vi "LaserLineDetection_Intensity_Imax.vi"(6 "Color":u32(colorbox)=16744448, 8 "error in (no error)":errorcluster, 10 "Line Coordinates":i32[](array[numeric]), 11 "Image In":T2) -> (0 "error out":errorcluster, 1 "appended array":cluster{u8[], i32[]}[](array[cluster]), 2 "Point Information":T1, 3 "Image Out":T2)   [LabVIEW 2013]
uses:
  <vilib>/vision/Image Controls.llb/IMAQ Image.ctl
  Point Information.ctl
  <vilib>/vision/NI_Vision_Development_Module.lvlib
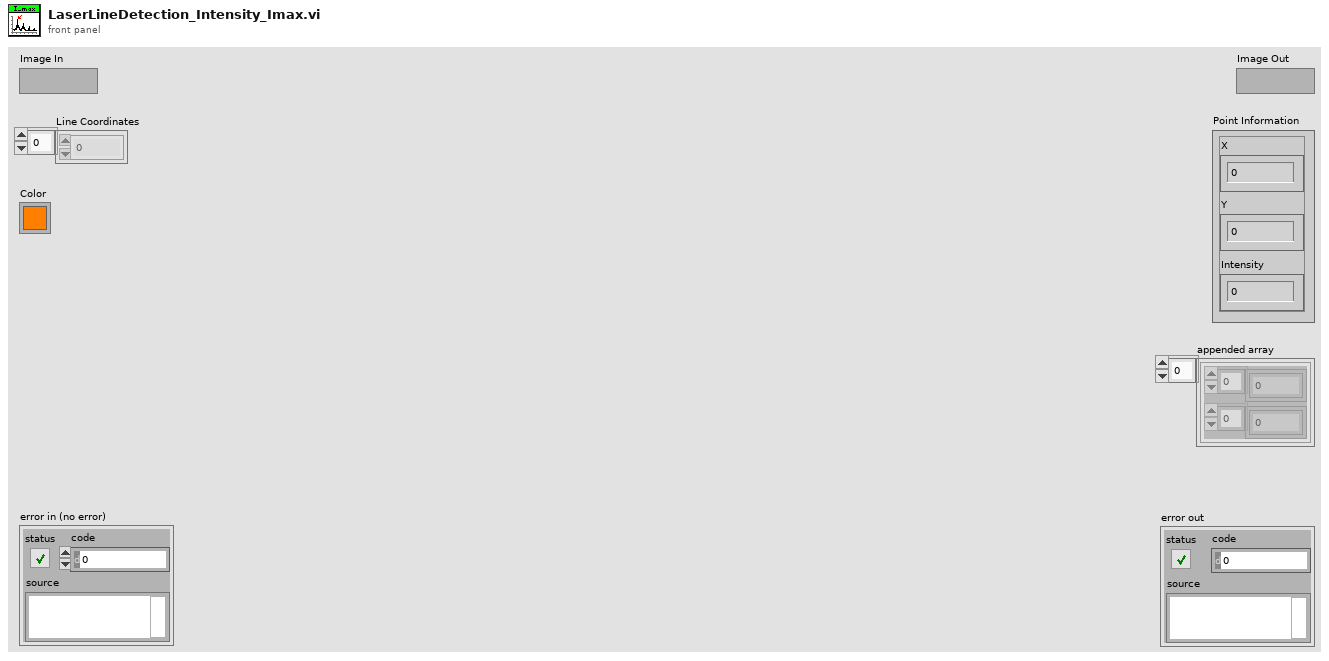
[diagram p1: front panel]
types:
  T1 = typedef "Point Information.ctl" = cluster{"X":i32, "Y":i32, "Intensity":u8}
  T2 = typedef "IMAQ Image.ctl" = refnum<image>
  T3 = cluster{"Red (or Hue) value":u8, "Green (or Sat) value":u8, "Blue (or Light or Val) value":u8}[]
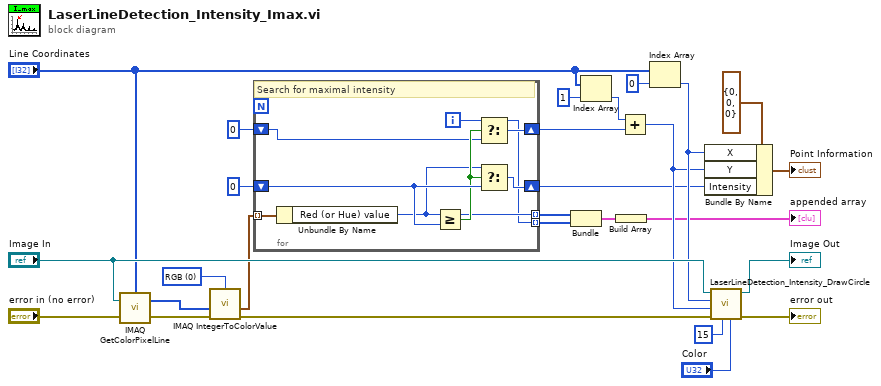
[diagram p0: block diagram]
diagram:
  w14 = u16 0 items=["RGB", "HSL", "HSV", "HSI"] ("Color Mode")
  n1 = call "IMAQ GetColorPixelLine"("Line Coordinates"="Line Coordinates", "Image"="Image In", "error in (no error)"="error in (no error)") -> ("Pixels Line (U32)"=w16:u32[], "error out"=w15:errorcluster)  [unwired: 1 in, 1 out]
  n2 = call "IMAQ IntegerToColorValue"("error in (no error)"=w15, "1D U32 array"=w16, "Color Mode"=w14) -> ("1D Color value array"=w17:T3, "error out"=w22:errorcluster)  [unwired: 2 in, 2 out]
  n3 = for {
    tunnel: w17 -> [w35] mode=indexing
    shift-right: [w33] -> w7
    shift-left: u8 0 ("y") -> [w34]
    shift-right: [w30] -> w24
    shift-left: 0 ("Y_center") -> [w31]
    tunnel: [w29] -> w4 mode=indexing
    tunnel: [w28] -> w1 mode=indexing
    i -> [w28]
    # "Search for maximal intensity"
    n4 = Unbundle By Name(w35) -> ("Red (or Hue) value"=w29:u8)
    n5 = Greater Or Equal?(x=w29, y=w34) -> (x >= y?=w32:bool)
    n6 = Select(t=w28, s=w32, f=w31) -> (s? t:f=w30:i32)
    n7 = Select(t=w29, s=w32, f=w34) -> (s? t:f=w33:u8)
  }
  n8 = Bundle(w4, w1) -> (w3:cluster{u8[], i32[]})  [unwired: 1 in]
  n9 = Index Array(array="Line Coordinates", index=1) -> (element=w25:i32)
  n10 = Build Array(w3) -> (→"appended array":cluster{u8[], i32[]}[])
  n11 = Add(x=w25, y=w24) -> (x+y=w8:i32)
  n12 = Index Array(array="Line Coordinates", index=0) -> (element=w9:i32)
  n13 = Bundle By Name(cluster=T1 {"X"=0, "Y"=0, "Intensity"=0} ("Point Information"), "X"=w9, "Y"=w8, "Intensity"=w7) -> (→"Point Information":T1)
  n14 = call "LaserLineDetection_Intensity_DrawCircle.vi"("Color"="Color", "Radius"=15, "Error In"=w22, "Y_center"=w8, "X_center"=w9, "Image in"="Image In") -> ("Error Out"=→"error out":errorcluster, "Image out"=→"Image Out":T2)  [unwired: 4 in]
